vi "read_attributes.vi"(8 "error in (no error)":errorcluster, 11 "TruncatedSVD in":refnum<class "TruncatedSVD.lvclass">) -> (0 "error out":errorcluster, 2 "attributes":T1, 3 "TruncatedSVD out":refnum<class "TruncatedSVD.lvclass">)   [LabVIEW 2020, in "TruncatedSVD.lvclass"]
uses:
  TruncatedSVD.lvclass
  Controls/truncated_svd_attributes.ctl
  TruncatedSVD.lvclass/TruncatedSVD.ctl
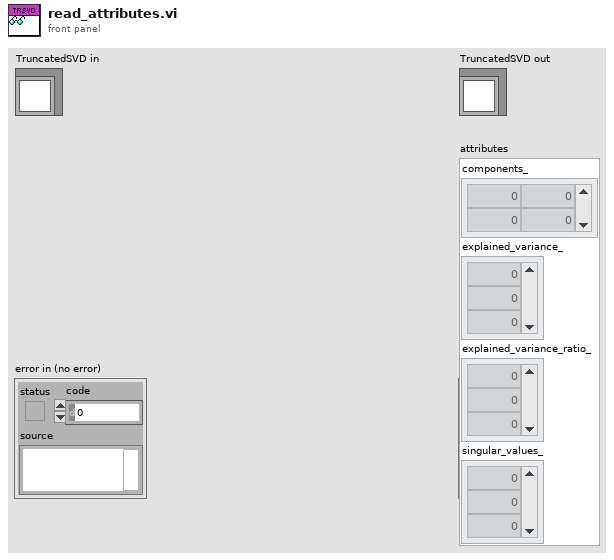
[diagram p1: front panel]
types:
  T1 = typedef "truncated_svd_attributes.ctl" = cluster{"components_":dbl[][], "explained_variance_":dbl[], "explained_variance_ratio_":dbl[], "singular_values_":dbl[]}
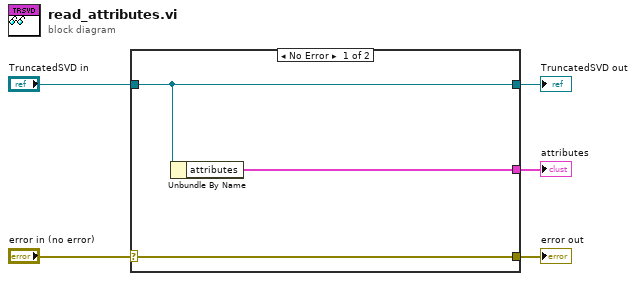
[diagram p0: block diagram]
diagram:
  n1 = case shown="No Error" "error in (no error)" {
    selector: "error in (no error)" -> [w8 w9]
    tunnel: [w8 w9] -> w4
    tunnel: [w7 w10] -> w2
    tunnel: "TruncatedSVD in" -> [w7 w10]
    tunnel: [w6 _] -> w1
    frame No Error {
      n2 = Unbundle By Name(w7) -> ("attributes"=w6:T1)
    }
    frame Error {
    }
  }
  "error out" <- w4
  "TruncatedSVD out" <- w2
  "attributes" <- w1
